vi "CheckBaxterEnabled.vi"(0 "error in":errorcluster, 3 "node":string) -> (1 "error out":errorcluster)   [LabVIEW 2012]
doc: "Check whether or not Baxter is enabled, and enables if Baxter is not"
uses:
  <userlib>/ROSforLV/ROS/Code/SubVIs/BaxterSide.ctl
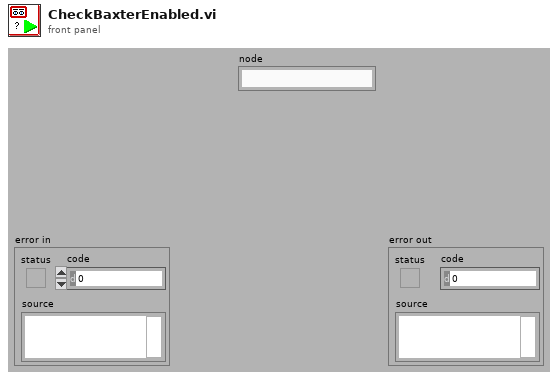
[diagram p1: front panel]
types:
  T1 = cluster{"Enabled?":bool, "Emergency Stop?":bool, "Component Error?":bool}
  T2 = typedef "BaxterSide.ctl" = enum16{"left", "right"}
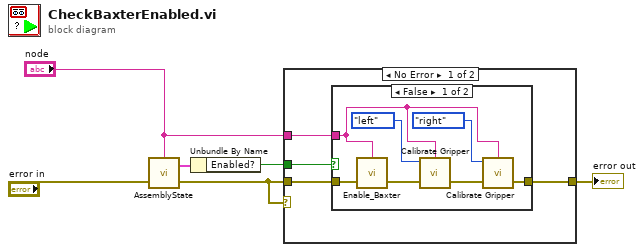
[diagram p0: block diagram]
diagram:
  n1 = call <userlib>:"AssemblyState.vi"("error in"="error in", "node"="node") -> ("error out"=w2:errorcluster, "Assembly State"=w5:T1)  [unwired: 1 in]
  n2 = Unbundle By Name(w5) -> ("Enabled?"=w6:bool)
  n3 = case shown="No Error" w2 {
    tunnel: w6 -> [w10 _]
    tunnel: w2 -> [w9 w19]
    tunnel: "node" -> [w8 _]
    tunnel: [w7 w19] -> w1
    frame No Error {
      n4 = case shown="False" w10 {
        tunnel: w9 -> [w13 w18]
        tunnel: [w11 w18] -> w7
        tunnel: w8 -> [w12 _]
        frame False {
          n5 = call <userlib>:"Enable_Baxter.vi"("error in"=w13, "node"=w12) -> ("error out"=w17:errorcluster)  [unwired: 2 in]
          n6 = call <userlib>:"Calibrate Gripper.vi"("node"=w12, "Side"=BaxterSide."left", "error in"=w17) -> ("error out"=w15:errorcluster)  [unwired: 3 in]
          n7 = call <userlib>:"Calibrate Gripper.vi"("node"=w12, "Side"=BaxterSide."right", "error in"=w15) -> ("error out"=w11:errorcluster)  [unwired: 3 in]
        }
        frame True {
        }
      }
    }
    frame Error {
    }
  }
  "error out" <- w1
